vi "Config Pulse Modulation.vi"(0 "VISA Resource Name":refnum<visa-resource-name>, 1 "PM Rate (400.0)":dbl=400.0 format="%.1f", 2 "Pulse Period (80.0)":dbl=80.0 format="%.1f", 3 "Pulse Width (40.0)":dbl=40.0 format="%.1f", 5 "Status (T:ON)":bool=TRUE, 7 "Pulse Source (0:Internal)":enum16{"INTERNAL", "EXT1", "EXT2"}(ring), 9 "Waveform (F:PULSE)":bool, 11 "error in (no error)":errorcluster {"code" format="%.0x"}) -> (4 "VISA Resource Name Out":refnum<visa-resource-name>, 15 "error out":errorcluster {"code" format="%.0x"})   [LabVIEW 2014, in "Agilent ESG Series.lvlib"]
doc: "This VI is used to set the modulation controls and the parameters associated with pulse modulated signals."
uses:
  Agilent ESG Series.lvlib
panel:
  # "SQUARE"
  # "PULSE"
  # "ON"
  # "OFF"
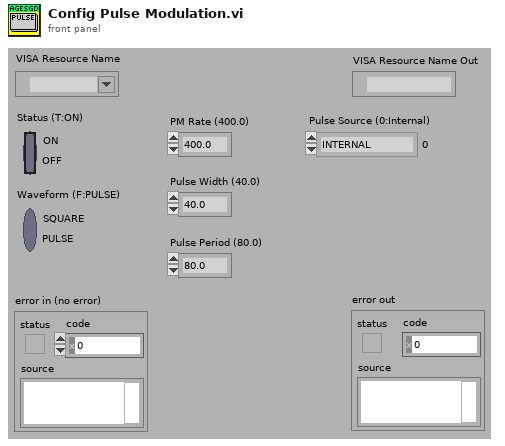
[diagram p1: front panel]
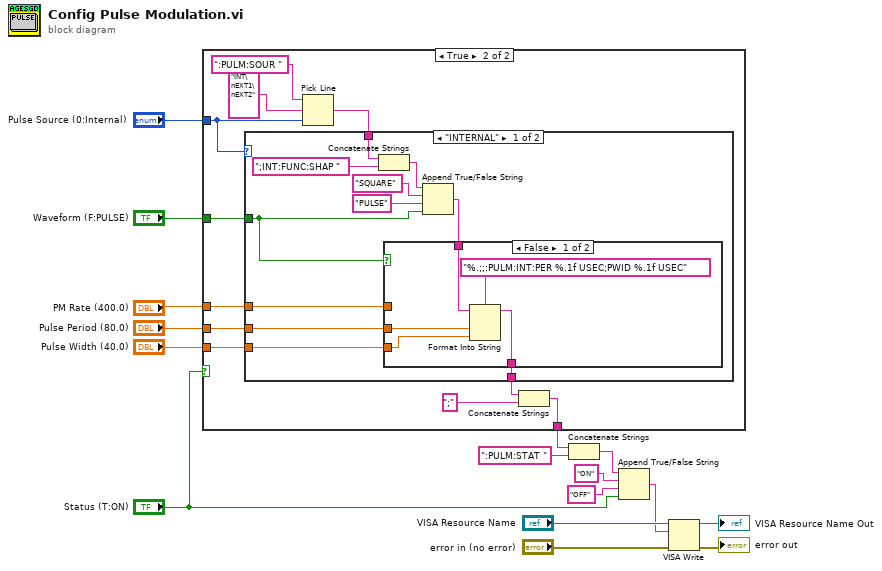
[diagram p0: block diagram]
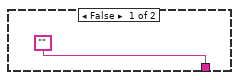
[diagram p2: hidden frame]
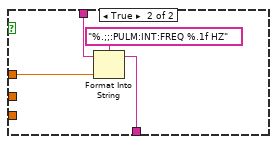
[diagram p3: hidden frame]
diagram:
  n1 = case shown="True" "Status (T:ON)" {
    tunnel: "Waveform (F:PULSE)" -> [_ w28]
    tunnel: "Pulse Width (40.0)" -> [_ w27]
    tunnel: ["" w19] -> w4
    tunnel: "Pulse Source (0:Internal)" -> [_ w26]
    tunnel: "Pulse Period (80.0)" -> [_ w22]
    tunnel: "PM Rate (400.0)" -> [_ w21]
    frame False {
    }
    frame True {
      n2 = Pick Line(string ("")=":PULM:SOUR ", multi-line string="INT\nEXT1\nEXT2", line index=w26) -> (output string=w23:string)
      n3 = case shown="\"INTERNAL\"" w26 {
        tunnel: w23 -> [w30 w49]
        tunnel: [w37 w49] -> w20
        tunnel: w21 -> [w32 _]
        tunnel: w22 -> [w38 _]
        tunnel: w27 -> [w35 _]
        tunnel: w28 -> [w34 _]
        frame "INTERNAL" {
          n4 = Concatenate Strings(w30, ";INT:FUNC:SHAP ") -> (w31:string)
          n5 = Append True/False String(1:w34, 2:"PULSE" ("false string"), 3:"SQUARE" ("true string"), 4:w31) -> (0:w33:string)
          n6 = case shown="False" w34 {
            tunnel: w35 -> [w44 _]
            tunnel: [w42 w45] -> w37
            tunnel: w38 -> [w41 _]
            tunnel: w33 -> [w40 w47]
            tunnel: w32 -> [_ w48]
            frame False {
              n7 = Format Into String(format string="%.;;:PULM:INT:PER %.1f USEC;PWID %.1f USEC", initial string=w40, w41, w44) -> (resulting string=w42:string)  [unwired: 1 in, 1 out]
            }
            frame True {
              n8 = Format Into String(format string="%.;;:PULM:INT:FREQ %.1f HZ", initial string=w47, w48) -> (resulting string=w45:string)  [unwired: 1 in, 1 out]
            }
          }
        }
        frame "EXT1", "EXT2" {
        }
      }
      n9 = Concatenate Strings(w20, ";" ("string")) -> (w19:string)
    }
  }
  n10 = Concatenate Strings(w4, ":PULM:STAT ") -> (w8:string)
  n11 = Append True/False String(1:"Status (T:ON)", 2:"OFF" ("false string"), 3:"ON" ("true string"), 4:w8) -> (0:w10:string)
  n12 = VISA Write(VISA resource name="VISA Resource Name", write buffer=w10, error in (no error)="error in (no error)") -> (VISA resource name out=→"VISA Resource Name Out":refnum<visa-resource-name>, error out=→"error out":errorcluster)  [unwired: 1 out]
